vi "LVCAM Write Self Actor.vi"(10 "Self Actor":refnum<class "LVCAM.lvclass">, 11 "LVCAM Write Self Actor in":refnum<class "LVCAM Write Self Actor.lvclass">) -> (3 "LVCAM Write Self Actor out":refnum<class "LVCAM Write Self Actor.lvclass">)   [LabVIEW 2021, in "LVCAM.lvlib" / "LVCAM Write Self Actor.lvclass"]
uses:
  LVCAM Write Self Actor.lvclass
  LVCAM/LVCAM.lvclass
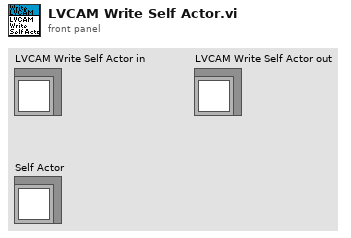
[diagram p1: front panel]
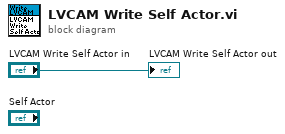
[diagram p0: block diagram]
diagram:
  "LVCAM Write Self Actor out" <- "LVCAM Write Self Actor in"
